vi "Fix Custom Device Order.vi"(8 "error in":errorcluster, 11 "Device Item Ref in":T1 format="%.0x") -> (0 "error out":errorcluster, 3 "Device Item Ref out":T1 format="%.0x")   [LabVIEW 2020, in "Routing and Faulting System Explorer.lvlib"]
uses:
  Routing and Faulting System Explorer.lvlib
  <vilib>/NI VeriStand/Custom Device API/Custom Device Item Ref.ctl
  <vilib>/NI VeriStand/Custom Device API/Custom Device API.lvlib
  Shared/Routing and Faulting Hardware API/Routing and Faulting Hardware API.lvlib
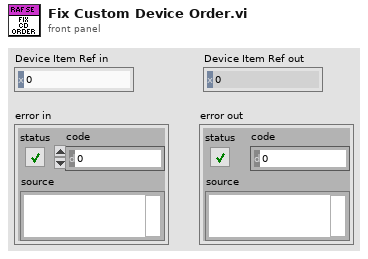
[diagram p1: front panel]
types:
  T1 = typedef "Custom Device API.lvlib/Custom Device Item Ref.ctl" = u64
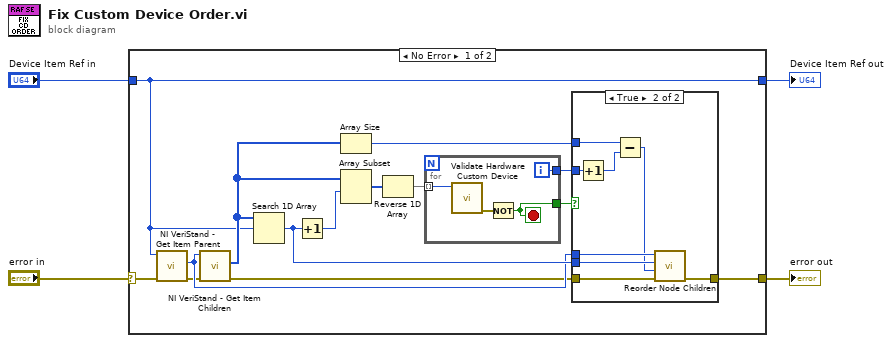
[diagram p0: block diagram]
diagram:
  n1 = case shown="No Error" "error in" {
    selector: "error in" -> [w8 w33]
    tunnel: [w16 w33] -> w4
    tunnel: "Device Item Ref in" -> [w5 w32]
    tunnel: [w5 w32] -> w1
    frame No Error {
      n2 = call <vilib>:"NI VeriStand - Get Item Parent.vi"("error in (no error)"=w8, "Item Ref in"=w5) -> ("error out"=w7:errorcluster, "Parent Ref"=w17:T1)  [unwired: 6 in, 2 out]
      n3 = call <vilib>:"NI VeriStand - Get Item Children.vi"("error in (no error)"=w7, "Item Ref in"=w17) -> ("error out"=w15:errorcluster, "Child Refs"=w6:T1[])  [unwired: 6 in, 2 out]
      n4 = Search 1D Array(1D array=w6, element=w5) -> (index of element=w18:i32)  [unwired: 1 in]
      n5 = Increment(x=w18) -> (x+1=w10:i32)
      n6 = Array Size(array=w6) -> (size(s)=w12:i32)
      n7 = Array Subset(array=w6, index=w10) -> (w9:T1[])  [unwired: 1 in]
      n8 = Reverse 1D Array(array=w9) -> (reversed array=w11:T1[])
      n9 = for {
        tunnel: w11 -> [w31] mode=indexing
        tunnel: [w29] -> w14
        tunnel: [w28] -> w13
        i -> [w28]
        stop <- w29 stop-if-true
        n10 = call "Validate Hardware Custom Device.vi"("Hardware Ref in"=w31) -> ("error out"=w30:errorcluster)  [unwired: 9 in, 1 out]
        n11 = Not(x=w30) -> (.not. x?=w29:bool)
      }
      n12 = case shown="True" w14 {
        tunnel: w12 -> [_ w27]
        tunnel: w13 -> [_ w26]
        tunnel: w15 -> [w19 w24]
        tunnel: [w19 w23] -> w16
        tunnel: w17 -> [_ w22]
        tunnel: w18 -> [_ w21]
        frame False {
        }
        frame True {
          n13 = Increment(x=w26) -> (x+1=w25:i32)
          n14 = Subtract(x=w27, y=w25) -> (x-y=w20:i32)
          n15 = call "Reorder Node Children.vi"("error in"=w24, "new index"=w20, "current index"=w21, "parent section in"=w22) -> ("error out"=w23:errorcluster)  [unwired: 7 in]
        }
      }
    }
    frame Error {
    }
  }
  "error out" <- w4
  "Device Item Ref out" <- w1
